vi "Create x-y Graph_Tilt Table.vi"(8 "Number of Elements (n)":i32=200, 9 "Time Step (s)":dbl=0.05, 10 "Reset":bool, 11 "Data In":dbl[](array[numeric])) -> (3 "XY Graph":cluster{dbl[], "Buffer Out":sgl[]}[](array[cluster]))   [LabVIEW 2014]
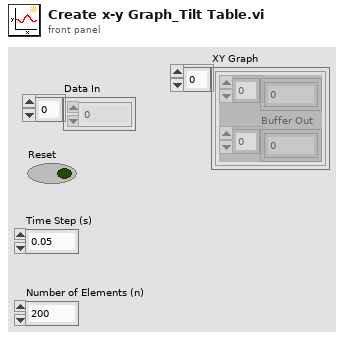
[diagram p1: front panel]
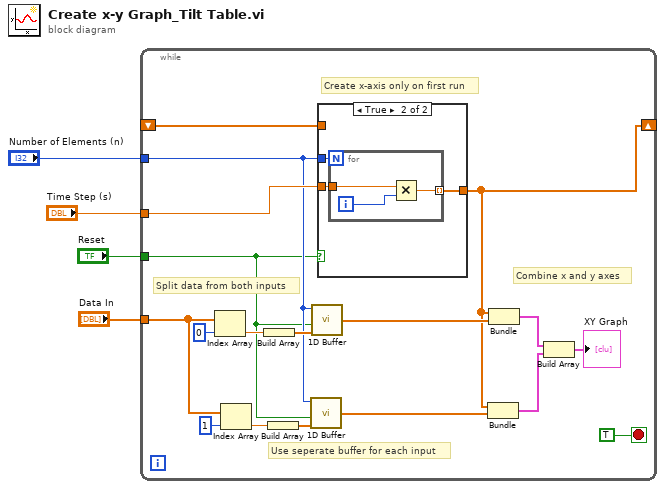
[diagram p0: block diagram]
diagram:
  n1 = while {
    tunnel: "Reset" -> [w6]
    tunnel: "Data In" -> [w14]
    shift-right: [w7] -> _
    shift-left: _ -> [w5]
    tunnel: "Time Step (s)" -> [w9]
    tunnel: "Number of Elements (n)" -> [w8]
    stop <- TRUE stop-if-true
    # "Combine x and y axes"
    # "Use seperate buffer for each input"
    # "Split data from both inputs"
    # "Create x-axis only on first run"
    n2 = Index Array(array=w14, index=0) -> (element=w18:dbl)
    n3 = Index Array(array=w14, index=1) -> (element=w21:dbl)
    n4 = Build Array(w18) -> (w19:dbl[])
    n5 = Build Array(w21) -> (w22:dbl[])
    n6 = call "1D Buffer.vi"("Data In"=w22, "Reset"=w6, "buffer size"=w8) -> ("Buffer Out"=w20:sgl[])  [unwired: 1 in]
    n7 = call "1D Buffer.vi"("Data In"=w19, "Reset"=w6, "buffer size"=w8) -> ("Buffer Out"=w17:sgl[])  [unwired: 1 in]
    n8 = case shown="True" w6 {
      tunnel: w9 -> [_ w26]
      tunnel: w8 -> [_ w25]
      tunnel: [w23 w24] -> w7
      tunnel: w5 -> [w23 _]
      frame False {
      }
      frame True {
        n9 = for {
          N: w25 -> [_]
          tunnel: [w28] -> w24 mode=indexing
          tunnel: w26 -> [w27]
          i -> [w29]
          n10 = Multiply(x=w27, y=w29) -> (x*y=w28:dbl)
        }
      }
    }
    n11 = Bundle(w7, "Buffer Out"=w20) -> (w16:cluster{dbl[], "Buffer Out":sgl[]})  [unwired: 1 in]
    n12 = Bundle(w7, "Buffer Out"=w17) -> (w15:cluster{dbl[], "Buffer Out":sgl[]})  [unwired: 1 in]
    n13 = Build Array(w15, w16) -> (→"XY Graph":cluster{dbl[], "Buffer Out":sgl[]}[])
  }
